vi "VG-check_plot_selection.vi"(10 "data format Last":T1, 11 "data format":T1) -> (3 "data format out":T1)   [LabVIEW 2020, in "VG-VNA_GUI.lvlib" / "VG-VNA_GUI.lvclass"]
uses:
  VG-VNA_GUI.lvclass
  VG-data_format_selector.ctl
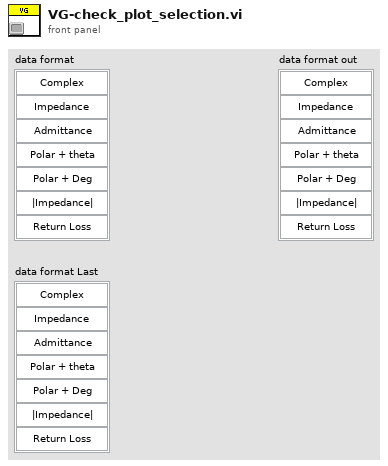
[diagram p1: front panel]
types:
  T1 = typedef "VG-VNA_GUI.lvlib/VG-VNA_GUI.lvclass/VG-data_format_selector.ctl" = cluster{"Complex":bool, "Impedance":bool, "Admittance":bool, "Polar":bool, "Polar Deg":bool, "|Impedance|":bool, "Return Loss":bool}
  T2 = cluster{"[0]":bool, "[1]":bool, "[2]":bool, "[3]":bool, "[4]":bool, "[5]":bool, "[6]":bool}
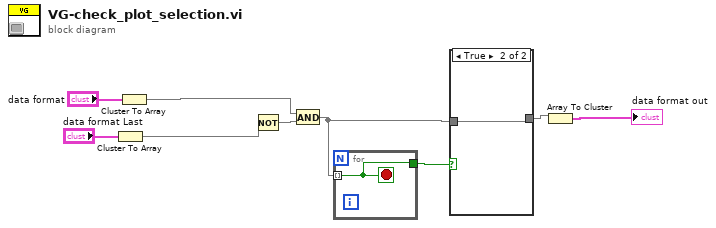
[diagram p0: block diagram]
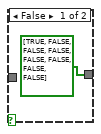
[diagram p2: hidden frame]
diagram:
  n1 = Cluster To Array(cluster="data format Last") -> (array=w1:bool[])
  n2 = Cluster To Array(cluster="data format") -> (array=w8:bool[])
  n3 = Not(x=w1) -> (.not. x?=w7:bool[])
  n4 = And(x=w8, y=w7) -> (x .and. y?=w5:bool[])
  n5 = for {
    tunnel: w5 -> [w10] mode=indexing
    tunnel: [w10] -> w6
    stop <- w10 stop-if-true
  }
  n6 = case shown="True" w6 {
    tunnel: w5 -> [_ w12]
    tunnel: [bool[] [TRUE, FALSE, FALSE, FALSE, FALSE, FALSE, FALSE, FALSE] w12] -> w4
    frame False {
    }
    frame True {
    }
  }
  n7 = Array To Cluster(array=w4) -> (cluster=→"data format out":T2)
